vi "9209_UI.vi"(8 "error in (no error)":errorcluster, 11 "Node Ptr":T1 format="%.0x") -> (0 "error out":errorcluster)   [LabVIEW 2017, in "Modules.lvlib" / "9209.lvclass"]
uses:
  9209.lvclass
  <vilib>/NI Veristand/Custom Device API/Custom Device Item Ref.ctl
  RSI Module/SubPanel Command.ctl
  C:/Users/nitest/Documents/ni-official/niveristand-scan-engine-module-libraries/Source/RSI Module/RSI Module.lvclass
  9209.lvclass/9209.ctl
  RSI Module/RSI Module.lvclass
  9205/9205.lvclass
  <vilib>/NI Veristand/Custom Device API/Custom Device API.lvlib
panel:
  in  "Conversion time":u32(ring) items=["High Speed", "High Resolution"]
  in  "_Update Chan Settings":bool
  in  "_Update Ring Controls":bool
  in  "_Terminal Modes":enum8{"RSE", "DIFF"}[](array[ring])=[enum."RSE", enum."RSE", enum."RSE", enum."RSE", enum."RSE", enum."RSE", enum."RSE", enum."RSE", enum."RSE", enum."RSE", enum."RSE", enum."RSE", enum."RSE", enum."RSE", enum."RSE", enum."RSE", enum."RSE", enum."RSE", enum."RSE", enum."RSE", enum."RSE", enum."RSE", enum."RSE", enum."RSE", enum."RSE", enum."RSE", enum."RSE", enum."RSE", enum."RSE", enum."RSE", enum."RSE", enum."RSE"]
  out "_SupportedTerminalModes":string[][](array[string])=[["RSE", "NRSE", "DIFF"], ["RSE", "NRSE", "DIFF"], ["RSE", "NRSE", "DIFF"], ["RSE", "NRSE", "DIFF"], ["RSE", "NRSE", "DIFF"], ["RSE", "NRSE", "DIFF"], ["RSE", "NRSE", "DIFF"], ["RSE", "NRSE", "DIFF"], ["RSE", "NRSE", ""], ["RSE", "NRSE", ""], ["RSE", "NRSE", ""], ["RSE", "NRSE", ""], ["RSE", "NRSE", ""], ["RSE", "NRSE", ""], ["RSE", "NRSE", ""], ["RSE", "NRSE", ""], ["RSE", "NRSE", "DIFF"], ["RSE", "NRSE", "DIFF"], ["RSE", "NRSE", "DIFF"], ["RSE", "NRSE", "DIFF"], ["RSE", "NRSE", "DIFF"], ["RSE", "NRSE", "DIFF"], ["RSE", "NRSE", "DIFF"], ["RSE", "NRSE", "DIFF"], ["RSE", "NRSE", ""], ["RSE", "NRSE", ""], ["RSE", "NRSE", ""], ["RSE", "NRSE", ""], ["RSE", "NRSE", ""], ["RSE", "NRSE", ""], ["RSE", "NRSE", ""], ["RSE", "NRSE", ""]]
  in  "Terminal Mode":u16(ring) items=["RSE", "DIFF"]
  in  "Channels":i32[](listbox)=[0]
  in  "SubPanel Event":refnum<user-event>
  in  "Header":cluster{"Section Name":string}={"Section Name"="NI 9209 Settings"}
  # "Channel Configuration"
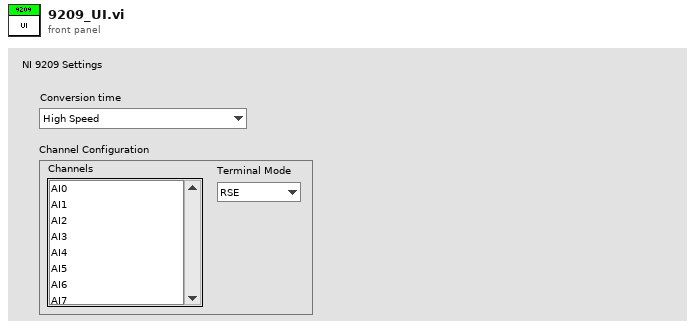
[diagram p1: front panel]
types:
  T1 = typedef "Custom Device API.lvlib/Custom Device Item Ref.ctl" = u64
  T2 = typedef "Modules.lvlib/9209.lvclass/Channel Settings.ctl" = T3[]
  T3 = typedef "Modules.lvlib/9209.lvclass/Terminal mode.ctl" = enum16{"RSE", "DIFF"}
  T4 = typedef "Modules.lvlib/RSI Module.lvclass/Module Models.ctl" = enum16{"Empty", "NI 9201", "NI 9203", "NI 9205", "NI 9206", "NI 9207", "NI 9208", "NI 9209", "NI 9211", "NI 9212", "NI 9213", "NI 9214", "NI 9215", "NI 9217", "NI 9219", "NI 9220", "NI 9221", "NI 9222", "NI 9223", "NI 9225", "NI 9227", "NI 9229", "NI 9233", "NI 9234", "NI 9235", "NI 9236", "NI 9237", "NI 9239", "NI 9242", "NI 9244", "NI 9263", "NI 9264", "NI 9265", "NI 9266", "NI 9269", "NI 9375", "NI 9401", "NI 9402", "NI 9403", "NI 9411", "NI 9421", "NI 9422", "NI 9423", "NI 9425", "NI 9426", "NI 9435", "NI 9437", "NI 9472", "NI 9474", "NI 9475", "NI 9476", "NI 9477", "NI 9478", "NI 9481", "NI 9482", "NI 9485"}
  T5 = typedef "Modules.lvlib/RSI Module.lvclass/SubPanel Command.ctl" = enum16{"Stop"}
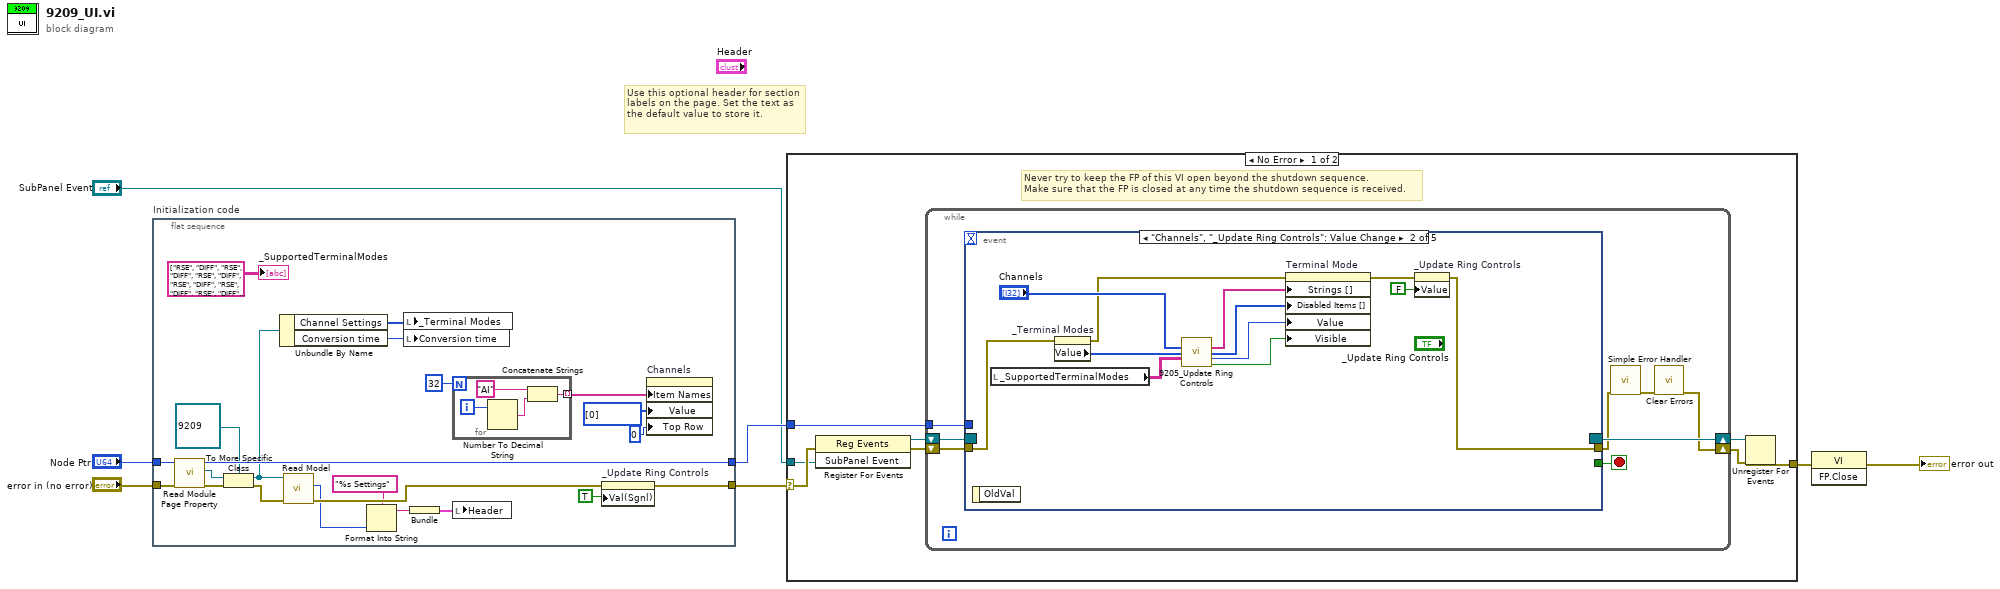
[diagram p0: block diagram]
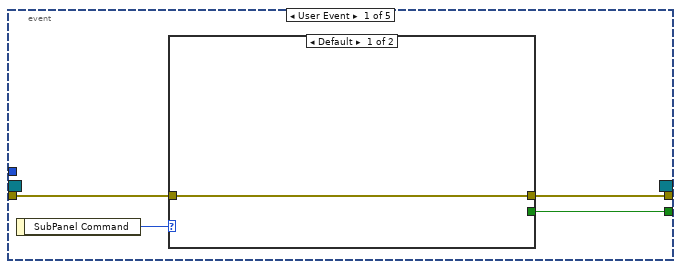
[diagram p2: hidden frame]
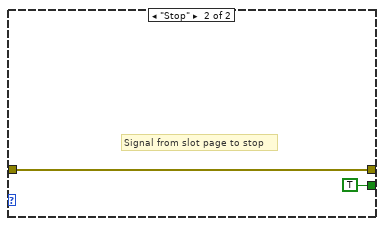
[diagram p3: hidden frame]
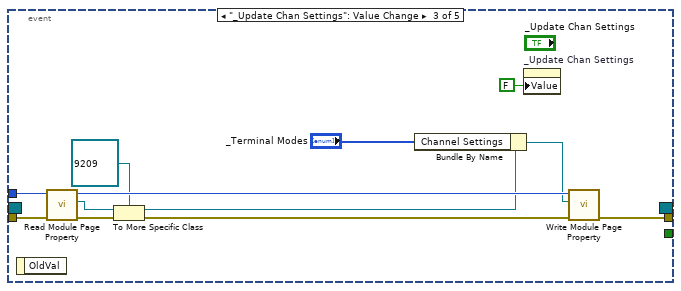
[diagram p4: hidden frame]
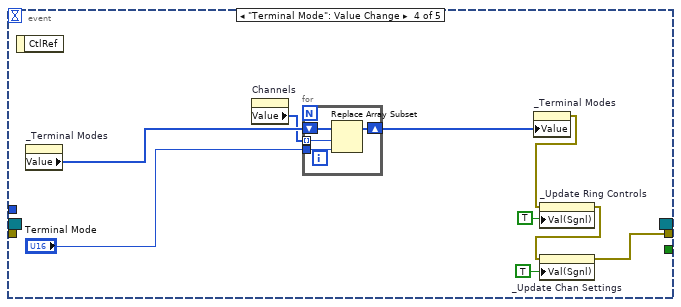
[diagram p5: hidden frame]
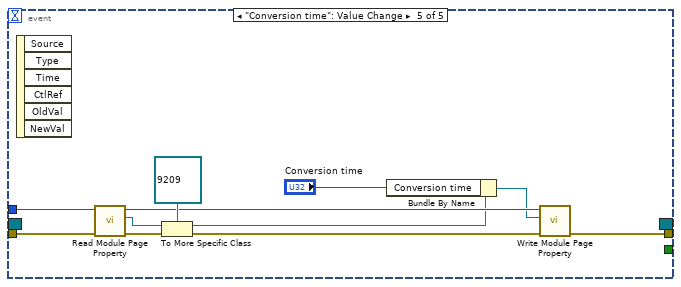
[diagram p6: hidden frame]
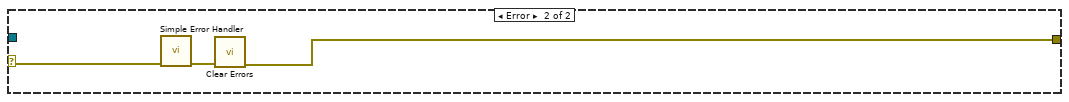
[diagram p7: hidden frame]
diagram:
  # "Use this optional header for section labels on the page. Set the text as the default value to store it."
  n1 = flat-sequence "Initialization code" {
    tunnel: "error in (no error)" -> [w28]
    tunnel: "Node Ptr" -> [w29]
    tunnel: [w22] -> w1
    tunnel: [w27] -> w4
    frame #0 {
      n2 = call "Read Module Page Property.vi"("error in (no error)"=w28, "Node Ptr In"=w29) -> ("error out"=w11:errorcluster, "RSI Module"=w10:refnum<class "RSI Module.lvclass">, "Node Ptr Out"=w27:T1)  [unwired: 7 in]
      n3 = To More Specific Class(target class=refnum<class "9209.lvclass"> refnum ("Modules.lvlib:9209.lvclass"), reference=w10, error in=w11) -> (specific class reference=w21:refnum<class "9209.lvclass">, error out=w9:errorcluster)
      n4 = Unbundle By Name(w21) -> ("Channel Settings"=w13:T2, "Conversion time"=w12:u32)
      n5 = call "Read Model.vi"("error in (no error)"=w9, "RSI Module in"=w21) -> ("error out"=w20:errorcluster, "Model"=w18:T4)  [unwired: 7 in, 1 out]
      n6 = Format Into String(format string="%s Settings", w18) -> (resulting string=w16:string)  [unwired: 2 in, 1 out]
      n7 = local write "_Terminal Modes"(w13) -> ()
      n8 = local write "Conversion time"(w12) -> ()
      n9 = Bundle(w16) -> (w19:cluster{string})  [unwired: 1 in]
      n10 = for {
        N: u32 32 ("NumChannels") -> [_]
        tunnel: [w30] -> w26 mode=indexing
        i -> [w32]
        n11 = Number To Decimal String(number=w32) -> (decimal integer string=w31:string)  [unwired: 1 out]
        n12 = Concatenate Strings("AI", w31) -> (w30:string)
      }
      n13 = local write "Header"(w19) -> ()
      n14 = property on="_Update Ring Controls" class="Bool (strict)"(error in=w20, "Val(Sgnl)"=TRUE ("Value (Signaling)")) -> (error out=w22:errorcluster)  [unwired: 1 in, 1 out]
      n15 = property on="Channels" class="LstBox (strict)"("Item Names"=w26, "Value"=i32[] [0] ("Channels"), "Top Row"=0) -> ()  [unwired: 2 in, 2 out]
      "_SupportedTerminalModes" <- string[][] [["RSE", "DIFF"], ["RSE", "DIFF"], ["RSE", "DIFF"], ["RSE", "DIFF"], ["RSE", "DIFF"], ["RSE", "DIFF"], ["RSE", "DIFF"], ["RSE", "DIFF"], ["RSE", ""], ["RSE", ""], ["RSE", ""], ["RSE", ""], ["RSE", ""], ["RSE", ""], ["RSE", ""], ["RSE", ""], ["RSE", "DIFF"], ["RSE", "DIFF"], ["RSE", "DIFF"], ["RSE", "DIFF"], ["RSE", "DIFF"], ["RSE", "DIFF"], ["RSE", "DIFF"], ["RSE", "DIFF"], ["RSE", ""], ["RSE", ""], ["RSE", ""], ["RSE", ""], ["RSE", ""], ["RSE", ""], ["RSE", ""], ["RSE", ""]] ("Terminal Modes")
    }
  }
  n16 = case shown="No Error" w1 {
    selector: w1 -> [w35 w107]
    tunnel: [w39 w105] -> w7
    tunnel: w4 -> [w36 _]
    tunnel: "SubPanel Event" -> [w34 _]
    frame No Error {
      # "Never try to keep the FP of this VI open beyond the shutdown sequence.\nMake sure that the FP is closed at any time the shutdown sequence is received."
      n17 = register-events(error in=w35, w34) -> (reference out=w37:refnum<event-registration>, error out=w38:errorcluster)  [unwired: 1 in]
      n18 = while {
        tunnel: w36 -> [w45]
        shift-right: [w42] -> w40
        shift-left: w38 -> [w48]
        shift-right: [w49] -> w41
        shift-left: w37 -> [w47]
        stop <- w46 stop-if-true
        n19 = event shown="[1] \"Channels\", \"_Update Ring Controls\": Value Change" {
          selector: w47 -> [_ _ _ _ _]
          dyn-events: [_ _ _ _ _] -> w49
          timeout: _ -> [_ _ _ _ _]
          tunnel: w48 -> [w52 w61 w75 _ w95]
          tunnel: [w51 _ _ _ _] -> w46
          tunnel: [w50 w58 w74 w86 w96] -> w44
          tunnel: w45 -> [_ _ w76 _ w94]
          event User Event {
            n20 = event-data() -> ("SubPanel Command"=w53:T5)  [unwired: 1 out]
            n21 = case shown="Default" w53 {
              tunnel: w52 -> [w54 w55]
              tunnel: [w54 w55] -> w50
              tunnel: [_ TRUE] -> w51
              frame Default {
              }
              frame "Stop" {
                # "Signal from slot page to stop"
              }
            }
          }
          event "Channels", "_Update Ring Controls": Value Change {
            n22 = event-data() -> ()  [unwired: 2 out]
            n23 = local read "_SupportedTerminalModes"() -> (w66:string[][])
            n24 = property on="_Terminal Modes" class="Arr (strict)"(error in=w61) -> (error out=w60:errorcluster, "Value"=w67:enum8{"RSE", "DIFF"}[])  [unwired: 1 in, 1 out]
            n25 = call "9205_Update Ring Controls.vi"("SelectedChannels"="Channels", "ChannelConfig"=w67, "SupportedModes"=w66) -> ("Strings out"=w57:string[], "Disabled Items out"=w65:i32[], "Value out"=w64:u8, "Visible out"=w63:bool)  [unwired: 9 in]
            n26 = property on="Terminal Mode" class="Ring (strict)"(error in=w60, "Strings []"=w57, "Disabled Items []"=w65, "Value"=w64, "Visible"=w63) -> (error out=w59:errorcluster)  [unwired: 1 in, 1 out]
            n27 = property on="_Update Ring Controls" class="Bool (strict)"(error in=w59, "Value"=FALSE ("_Update Ring Controls 2")) -> (error out=w58:errorcluster)  [unwired: 1 in, 1 out]
          }
          event "_Update Chan Settings": Value Change {
            n28 = event-data() -> ()  [unwired: 2 out]
            n29 = call "Read Module Page Property.vi"("error in (no error)"=w75, "Node Ptr In"=w76) -> ("error out"=w79:errorcluster, "RSI Module"=w80:refnum<class "RSI Module.lvclass">, "Node Ptr Out"=w77:T1)  [unwired: 7 in]
            n30 = To More Specific Class(target class=refnum<class "9209.lvclass"> refnum ("Modules.lvlib:9209.lvclass"), reference=w80, error in=w79) -> (specific class reference=w72:refnum<class "9209.lvclass">, error out=w78:errorcluster)
            n31 = Bundle By Name(cluster=w72, "Channel Settings"="_Terminal Modes") -> (w71:refnum<class "9209.lvclass">)
            n32 = property on="_Update Chan Settings" class="Bool (strict)"("Value"=FALSE ("_Update Values")) -> ()  [unwired: 2 in, 2 out]
            n33 = call "Write Module Page Property.vi"("error in (no error)"=w78, "RSI Module"=w71, "Node Ptr In"=w77) -> ("error out"=w74:errorcluster)  [unwired: 6 in, 2 out]
          }
          event "Terminal Mode": Value Change {
            n34 = event-data() -> ()  [unwired: 2 out]
            n35 = property on="_Terminal Modes" class="Arr (strict)"() -> ("Value"=w84:enum8{"RSE", "DIFF"}[])  [unwired: 2 in, 2 out]
            n36 = property on="Channels" class="LstBox (strict)"() -> ("Value"=w81:i32[])  [unwired: 2 in, 2 out]
            n37 = for {
              tunnel: "Terminal Mode" -> [w92]
              tunnel: w81 -> [w90] mode=indexing
              shift-right: [w91] -> w83
              shift-left: w84 -> [w93]
              n38 = Replace Array Subset(array=w93, new element=w92, index=w90) -> (w91:enum8{"RSE", "DIFF"}[])
            }
            n39 = property on="_Terminal Modes" class="Arr (strict)"("Value"=w83) -> (error out=w85:errorcluster)  [unwired: 2 in, 1 out]
            n40 = property on="_Update Ring Controls" class="Bool (strict)"(error in=w85, "Val(Sgnl)"=TRUE ("Value (Signaling)")) -> (error out=w87:errorcluster)  [unwired: 1 in, 1 out]
            n41 = property on="_Update Chan Settings" class="Bool (strict)"(error in=w87, "Val(Sgnl)"=TRUE ("Value (Signaling)")) -> (error out=w86:errorcluster)  [unwired: 1 in, 1 out]
          }
          event "Conversion time": Value Change {
            n42 = event-data() -> ()  [unwired: 7 out]
            n43 = call "Read Module Page Property.vi"("error in (no error)"=w95, "Node Ptr In"=w94) -> ("error out"=w102:errorcluster, "RSI Module"=w103:refnum<class "RSI Module.lvclass">, "Node Ptr Out"=w100:T1)  [unwired: 7 in]
            n44 = To More Specific Class(target class=refnum<class "9209.lvclass"> refnum ("9205 in"), reference=w103, error in=w102) -> (specific class reference=w99:refnum<class "9209.lvclass">, error out=w101:errorcluster)
            n45 = Bundle By Name(cluster=w99, "Conversion time"="Conversion time") -> (w98:refnum<class "9209.lvclass">)
            n46 = call "Write Module Page Property.vi"("error in (no error)"=w101, "RSI Module"=w98, "Node Ptr In"=w100) -> ("error out"=w96:errorcluster)  [unwired: 6 in, 2 out]
          }
        }
        n47 = call <vilib>:"Simple Error Handler.vi"("error in (no error)"=w44) -> ("error out"=w43:errorcluster)  [unwired: 1 in, 7 out]
        n48 = call <vilib>:"Clear Errors.vi"("error in (no error)"=w43) -> ("error out"=w42:errorcluster)  [unwired: 1 in, 5 out]
      }
      n49 = Unregister For Events(event registration refnum=w41, error in=w40) -> (error out=w39:errorcluster)
    }
    frame Error {
      n50 = call <vilib>:"Simple Error Handler.vi"("error in (no error)"=w107) -> ("error out"=w106:errorcluster)  [unwired: 1 in, 7 out]
      n51 = call <vilib>:"Clear Errors.vi"("error in (no error)"=w106) -> ("error out"=w105:errorcluster)  [unwired: 1 in, 5 out]
    }
  }
  n52 = invoke class="VI" method="FP.Close"(error in=w7) -> (error out=→"error out":errorcluster)  [unwired: 2 in, 2 out]
